vi "Picture_switch_value.vi"(8 "Boolean array in":bool[](array[boolean]), 10 "Value to switch":i32, 11 "Switch":bool) -> (0 "Boolean array out":bool[](array[boolean]), 2 "New Value":bool)   [LabVIEW 2009]
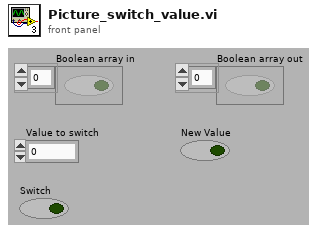
[diagram p1: front panel]
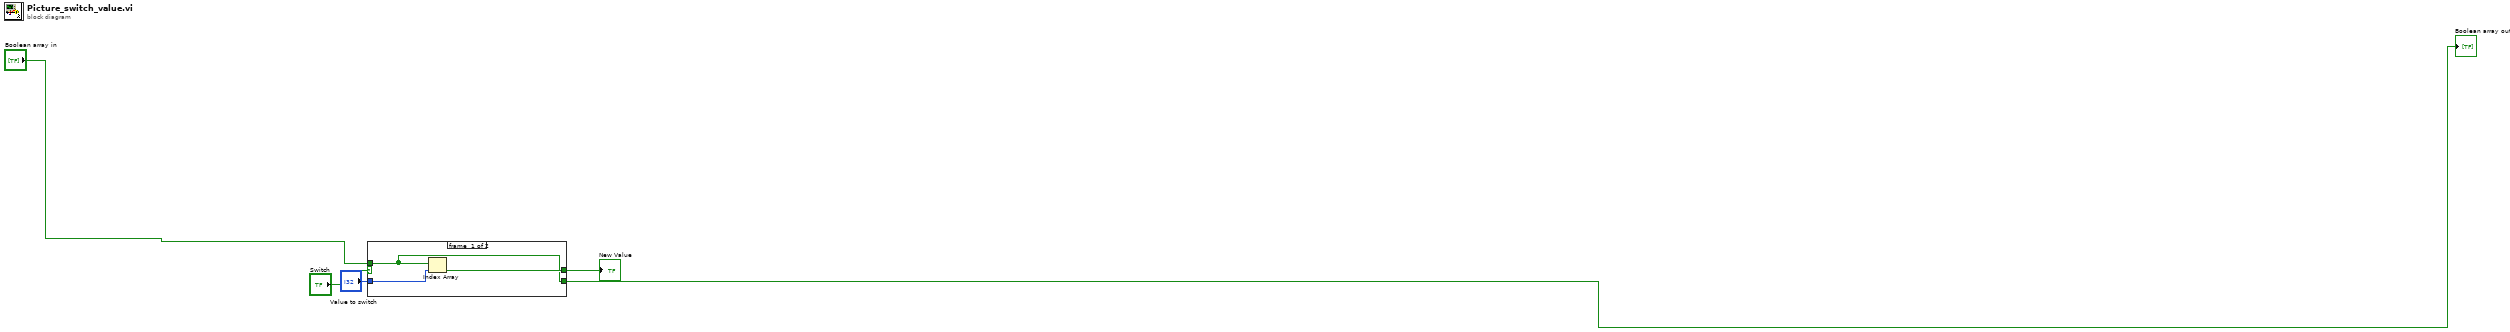
[diagram p0: block diagram]
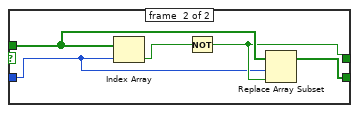
[diagram p2: hidden frame]
diagram:
  n1 = case shown="True" "Switch" {
    tunnel: "Boolean array in" -> [w7 w13]
    tunnel: [w8 w11] -> w4
    tunnel: [w7 w10] -> w1
    tunnel: "Value to switch" -> [w6 w9]
    frame #0 {
      n2 = Index Array(array=w7, index=w6) -> (element=w8:bool)
    }
    frame #1 {
      n3 = Index Array(array=w13, index=w9) -> (element=w12:bool)
      n4 = Not(x=w12) -> (.not. x?=w11:bool)
      n5 = Replace Array Subset(array=w13, new element=w11, index=w9) -> (w10:bool[])
    }
  }
  "New Value" <- w4
  "Boolean array out" <- w1
